vi "Release Relay Queues.vi"(8 "error in (no error)":errorcluster, 11 "queueIDList":string[](array[string])) -> (0 "error out":errorcluster)   [LabVIEW 2026, in "Tests.lvlib"]
doc: "Test teardown helper. Force-destroys the named relay queues for a set of appender ids, so no queue leaks into the process-global namespace between tests. Obtains each queue by its id-derived name (RelayQueueName, element type Statement) and releases it with force. A missing queue is a no-op, so it is safe to re-run and safe for ids whose queue was never created. Call after Shutdown has confirmed the manager stopped, so no appender can write into a destroyed queue."
uses:
  Tests.lvlib
  src/TypeDefs/Statement.ctl
  src/TypeDefs/Severity.ctl
  src/Lumberjack.lvlib
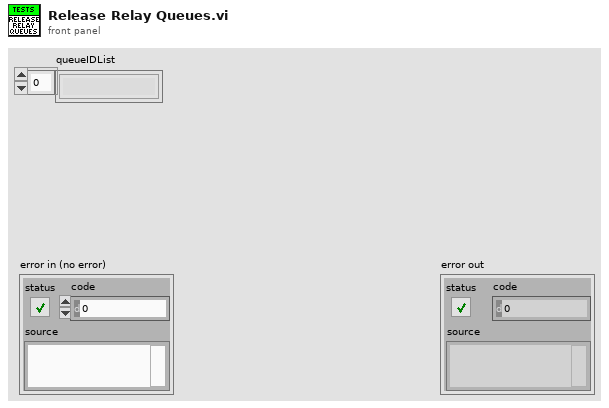
[diagram p1: front panel]
types:
  T1 = typedef "Lumberjack.lvlib/Statement.ctl" = cluster{"timestamp":timestamp, "level":T2, "sourceTag":string, "originVI":string, "message":string}
  T2 = typedef "Lumberjack.lvlib/Severity.ctl" = enum16{"OFF", "FATAL", "ERROR", "WARN", "INFO", "DEBUG", "TRACE", "ALL"}
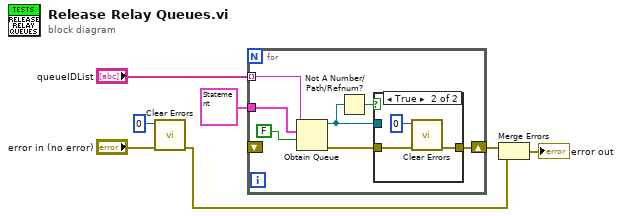
[diagram p0: block diagram]
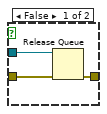
[diagram p2: hidden frame]
diagram:
  n1 = call <vilib>:"Clear Errors.vi"("error in (no error)"="error in (no error)", "specific error code to clear (0: all)"=0) -> ("error out"=w2:errorcluster)  [unwired: 4 in, 1 out]
  n2 = for {
    tunnel: "queueIDList" -> [w14] mode=indexing
    tunnel: T1 {"timestamp"=timestamp(0 s since 1904-01-01), "level"=enum."INFO", "sourceTag"="", "originVI"="", "message"=""} ("Statement") -> [w13]
    shift-right: [w11] -> w3
    shift-left: _ -> [_]
    n3 = Obtain Queue(name (unnamed)=w14, element data type=w13, create if not found? (T)=FALSE) -> (queue out=w9:refnum<queue>, error out=w10:errorcluster)  [unwired: 2 in, 1 out]
    n4 = Not A Number/Path/Refnum?(number/path/refnum=w9) -> (NaN/Path/Refnum?=w8:bool)
    n5 = case shown="True" w8 {
      tunnel: [w17 w18] -> w11
      tunnel: w10 -> [w16 w19]
      tunnel: w9 -> [w15 _]
      frame False {
        n6 = Release Queue(queue=w15, error in (no error)=w16) -> (error out=w17:errorcluster)  [unwired: 1 in, 2 out]
      }
      frame True {
        n7 = call <vilib>:"Clear Errors.vi"("error in (no error)"=w19, "specific error code to clear (0: all)"=0) -> ("error out"=w18:errorcluster)  [unwired: 4 in, 1 out]
      }
    }
  }
  n8 = Merge Errors(w3, w2) -> (→"error out":errorcluster)
